vi "Read.vi"(8 "error in (no error)":errorcluster, 11 "HAL.TCP in":refnum<class "HAL.TCP.lvclass">) -> (0 "error out":errorcluster, 2 "response":string, 3 "HAL.TCP out":refnum<class "HAL.TCP.lvclass">)   [LabVIEW 2019, in "HAL.TCP.lvclass"]
doc: "Override to <b>close</b> the connection to your hardware"
uses:
  HAL.TCP.lvclass
  HAL.TCP.lvclass/HAL.TCP.ctl
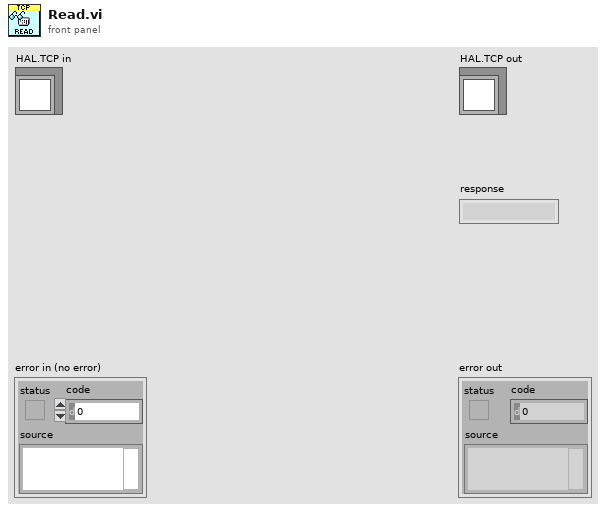
[diagram p1: front panel]
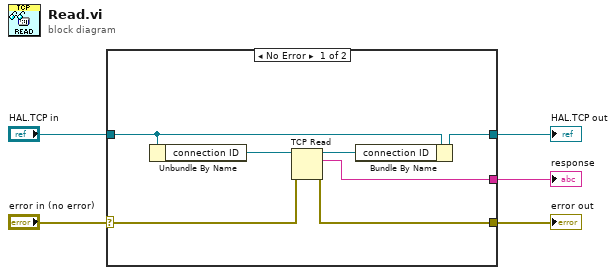
[diagram p0: block diagram]
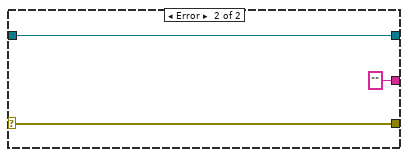
[diagram p2: hidden frame]
diagram:
  n1 = case shown="No Error" "error in (no error)" {
    selector: "error in (no error)" -> [w8 w15]
    tunnel: "HAL.TCP in" -> [w12 w14]
    tunnel: [w7 w15] -> w2
    tunnel: [w11 w14] -> w3
    tunnel: [w6 "" ("data out")] -> w1
    frame No Error {
      n2 = Unbundle By Name(w12) -> ("connection ID"=w10:refnum<k5>)
      n3 = TCP Read(connection ID=w10, error in (no error)=w8) -> (connection ID out=w9:refnum<k5>, data out=w6:string, error out=w7:errorcluster)  [unwired: 3 in]
      n4 = Bundle By Name(cluster=w12, "connection ID"=w9) -> (w11:refnum<class "HAL.TCP.lvclass">)
    }
    frame Error {
    }
  }
  "error out" <- w2
  "HAL.TCP out" <- w3
  "response" <- w1
